vi "GetPigeonIMU.vi"(8 "Reset Yaw (deg)":dbl format="%#_13g", 11 "Reset Yaw":bool) -> (0 "Yaw Rate (deg/s)":dbl format="%#_13g", 3 "Yaw (deg)":dbl format="%#_13g")   [LabVIEW 2020]
doc: "This VI reads the Pigeon IMU yaw, pitch, and roll values. It also handles error detection and orientation resets."
uses:
  refnumbers.vi
  <vilib>/Rock Robotics/WPI/ThirdParty/Phoenix-LabVIEW/Pigeon IMU/CTRE_PigeonIMU_GetRawGyro.vi
  <vilib>/Rock Robotics/WPI/ThirdParty/Phoenix-LabVIEW/Pigeon IMU/CTRE_PigeonIMU_GetYPR.vi
  sensordata.vi
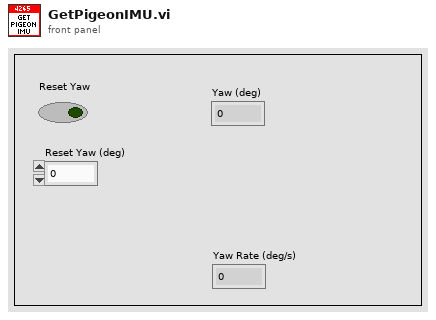
[diagram p1: front panel]
types:
  T1 = typedef "CTRE_PigeonIMU_DeviceRef.ctl" = cluster{"DeviceStatus":errorcluster, "Device Number":u8, "Type":T2, "Device ID":u32, "Handle":u64, "UsageFrame":u32, "Library Path":path}
  T2 = typedef "CTRE_PigeonIMU_ConnectionType.ctl" = u32
  T3 = cluster{"X":dbl, "Y":dbl, "Z":dbl, "Magnitude":dbl}
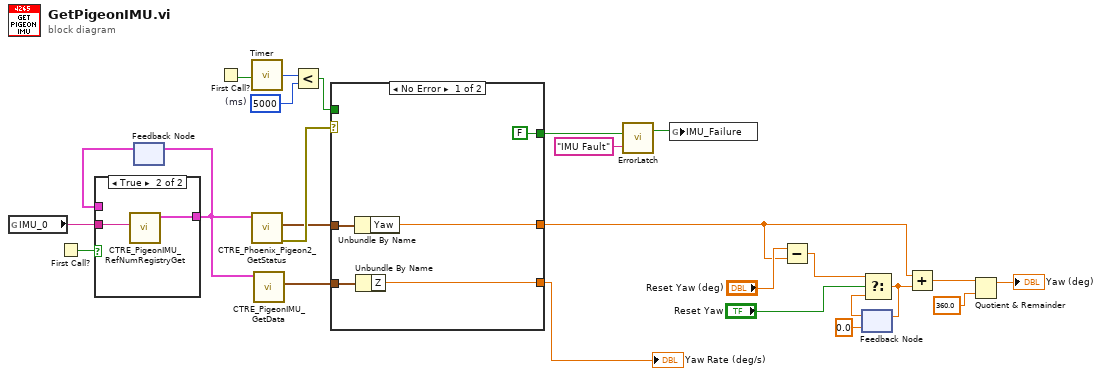
[diagram p0: block diagram]
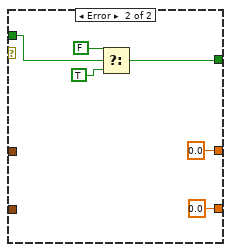
[diagram p2: hidden frame]
diagram:
  w6 = u32 5000  # (ms)
  n1 = global read "refnumbers.vi" "IMU_0"() -> (w24:string)
  n2 = First Call?() -> (First Call?: T/F=w11:bool)
  n3 = feedback #1() -> (w25:T1)  [unwired: 1 in]
  n4 = case shown="True" w11 {
    tunnel: [w26 w28] -> w2
    tunnel: w25 -> [w26 _]
    tunnel: w24 -> [_ w27]
    frame False {
    }
    frame True {
      n5 = call <vilib>:"CTRE_PigeonIMU_RefNumRegistryGet.vi"("refnum name"=w27) -> ("PigeonIMUDevRef"=w28:T1)  [unwired: 9 in, 1 out]
    }
  }
  n6 = feedback-in #1(w2) -> ()
  n7 = First Call?() -> (First Call?: T/F=w8:bool)
  n8 = call "Timer.vi"("Reset Timer"=w8) -> ("Time (ms)"=w7:u32)
  n9 = call-poly <vilib>:"CTRE_Phoenix_Pigeon2_GetStatus.vi"("PigeonIMUDevRef"=w2) -> ("error out"=w10:errorcluster, "Yaw Pitch Roll"=w9:cluster{"Yaw":dbl, "Pitch":dbl, "Roll":dbl})  [unwired: 8 in, 1 out]
  n10 = call-poly <vilib>:"CTRE_PigeonIMU_GetData.vi"("PigeonIMUDevRef"=w2) -> ("Gyro DPS"=w1:T3)  [unwired: 8 in, 2 out]
  n11 = Less?(x=w7, y=w6) -> (x < y?=w5:bool)
  n12 = case shown="No Error" w10 {
    tunnel: [FALSE w35] -> w15
    tunnel: w9 -> [w32 _]
    tunnel: [w31 0.0 ("Yaw")] -> w13
    tunnel: w5 -> [_ w38]
    tunnel: [w30 0.0 ("X")] -> w3
    tunnel: w1 -> [w29 _]
    frame No Error {
      n13 = Unbundle By Name(w32) -> ("Yaw"=w31:dbl)
      n14 = Unbundle By Name(w29) -> ("Z"=w30:dbl)
    }
    frame Error {
      n15 = Select(t=FALSE, s=w38, f=TRUE) -> (s? t:f=w35:bool)
    }
  }
  "Yaw Rate (deg/s)" <- w3
  n16 = call "ErrorLatch.vi"("Error Message"="IMU Fault", "Trigger"=w15) -> ("Latched"=w14:bool)  [unwired: 1 in]
  n17 = global write "sensordata.vi" "IMU_Failure"(w14) -> ()
  n18 = Subtract(x="Reset Yaw (deg)", y=w13) -> (x-y=w23:dbl)
  n19 = feedback #2(0.0) -> (w22:dbl)
  n20 = Select(t=w23, s="Reset Yaw", f=w22) -> (s? t:f=w20:dbl)
  n21 = feedback-in #2(w20) -> ()
  n22 = Add(x=w13, y=w20) -> (x+y=w17:dbl)
  n23 = Quotient & Remainder(x=w17, y=360.0) -> (x-y*floor(x/y)=→"Yaw (deg)":dbl)  [unwired: 1 out]
